vi "Get DAQmxTask_.vi"(8 "error in (no error)":errorcluster, 10 "Task name":string, 11 "DAQmxTaksContainer_General in":refnum<class "DAQmxTaksContainer_General.lvclass">) -> (0 "error out":errorcluster, 2 "DAQmx Task":refnum<class "DAQmxTask.lvclass">, 3 "DAQmxTaksContainer_General out":refnum<class "DAQmxTaksContainer_General.lvclass">)   [LabVIEW 2015, in "DAQmxTaksContainer_General.lvclass"]
uses:
  DAQmxTaksContainer_General.lvclass
  DAQmxTask.lvclass
  DAQmxTaksContainer_General.lvclass/DAQmxTaksContainer_General.ctl
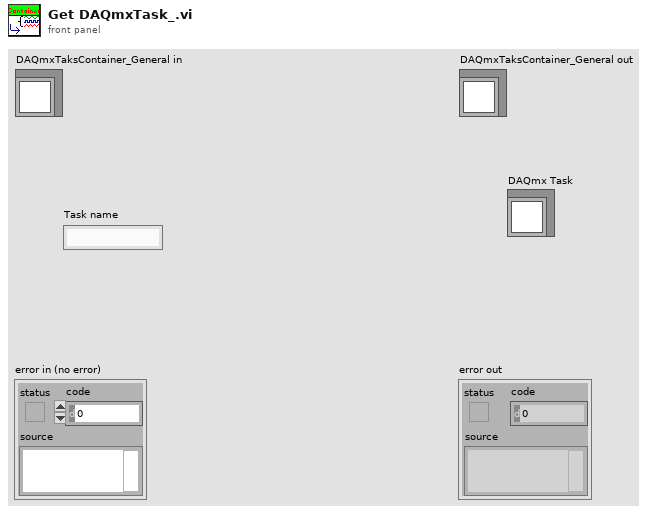
[diagram p1: front panel]
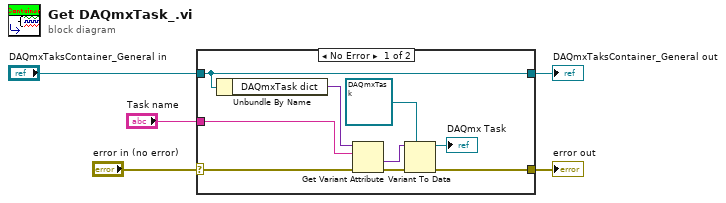
[diagram p0: block diagram]
diagram:
  n1 = case shown="No Error" "error in (no error)" {
    selector: "error in (no error)" -> [w11 w16]
    tunnel: [w8 w16] -> w3
    tunnel: [w14 w15] -> w4
    tunnel: "DAQmxTaksContainer_General in" -> [w14 w15]
    tunnel: "Task name" -> [w12 _]
    frame No Error {
      n2 = Unbundle By Name(w14) -> ("DAQmxTask dict"=w13:variant)
      n3 = Get Variant Attribute(Variant=w13, name=w12, error in=w11) -> (value=w10:variant, error out=w9:errorcluster)  [unwired: 1 in, 2 out]
      n4 = Variant To Data(error in=w9, type=refnum<class "DAQmxTask.lvclass"> refnum ("DAQmxTask.lvclass"), Variant=w10) -> (data=→"DAQmx Task":refnum<class "DAQmxTask.lvclass">, error out=w8:errorcluster)
    }
    frame Error {
    }
  }
  "error out" <- w3
  "DAQmxTaksContainer_General out" <- w4
